vi "poly_recursive_set_cluster_element(s).vi"(6 "stop after 1st one?":bool, 7 "delimiter (/)":string="/", 8 "error in (no error)":errorcluster, 9 "field name":string, 10 "Data":variant, 11 "Cluster":variant) -> (0 "error out":errorcluster, 2 "set?":bool, 3 "Cluster out":variant)   [LabVIEW 2015]
uses:
  <vilib>/Utility/Data Type/NI_Data Type.lvlib
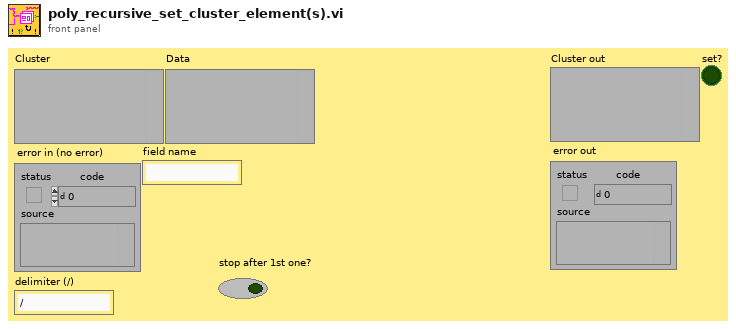
[diagram p1: front panel]
types:
  T1 = typedef "NI_Data Type.lvlib/Data Type.ctl" = enum8{"Invalid Type", "Void", "I8", "I16", "I32", "I64", "U8", "U16", "U32", "U64", "Single Float", "Double Float", "Extended Float", "Single Complex", "Double Complex", "Extended Complex", "Enum U8", "Enum U16", "Enum U32", "Enum U64", "Single Float With Unit", "Double Float With Unit", "Extended Float With Unit", "Single Complex with Unit", "Double Complex with Unit", "Extended Complex with Unit", "Boolean", "String", "Path", "Picture", "Tag", "Array", "Cluster", "Variant", "LV Variant", "Waveform", "Timestamp", "Digital Waveform", "Digital Data", "ExpressData", "Refnum", "External Data", "VI", "Poly VI", "LabVIEW Class Instance", "Fixed Point"}
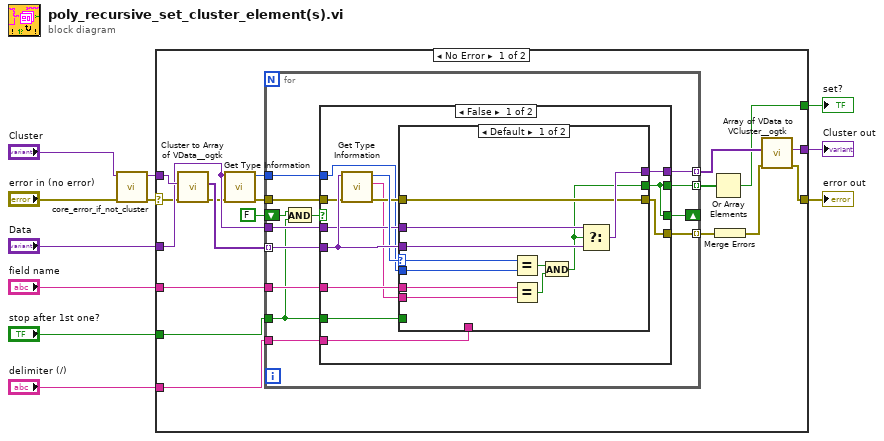
[diagram p0: block diagram]
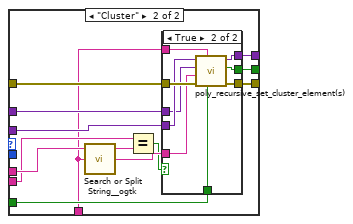
[diagram p2: hidden frame]
diagram:
  n1 = call "core_error_if_not_cluster.vi"("Error in"="error in (no error)", "Cluster"="Cluster") -> ("Error out"=w4:errorcluster, "Cluster duplicate"=w2:variant)  [unwired: 8 in]
  n2 = case shown="No Error" w4 {
    selector: w4 -> [w15 w94]
    tunnel: w2 -> [w28 _]
    tunnel: [w26 _] -> w11
    tunnel: "Data" -> [w17 _]
    tunnel: [w23 w94] -> w9
    tunnel: "field name" -> [w22 _]
    tunnel: [w20 _] -> w7
    tunnel: "stop after 1st one?" -> [w19 _]
    tunnel: "delimiter (/)" -> [w12 _]
    frame No Error {
      n3 = call <userlib>:"Cluster to Array of VData__ogtk.vi"("error in (no error)"=w15, "Cluster"=w28) -> ("error out"=w14:errorcluster, "Array of VData"=w29:variant[])  [unwired: 8 in]
      n4 = call <vilib>:"Get Type Information.vi"("error in (no error)"=w14, "Variant"=w17) -> ("error out"=w13:errorcluster, "Type"=w16:T1)  [unwired: 5 in, 3 out]
      n5 = for {
        tunnel: w29 -> [w41] mode=indexing
        tunnel: [w42] -> w27 mode=indexing
        tunnel: w17 -> [w40]
        tunnel: [w38] -> w25 mode=indexing
        tunnel: w13 -> [w39]
        tunnel: w22 -> [w37]
        tunnel: [w32] -> w21 mode=indexing
        shift-right: [w36] -> _
        shift-left: FALSE ("set?") -> [w34]
        tunnel: w19 -> [w31]
        tunnel: w16 -> [w35]
        tunnel: w12 -> [w30]
        n6 = And(x=w34, y=w31) -> (x .and. y?=w33:bool)
        n7 = case shown="False" w33 {
          selector: w33 -> [_ w92]
          tunnel: [w55 w91] -> w42
          tunnel: w41 -> [w54 w91]
          tunnel: w40 -> [w52 _]
          tunnel: w39 -> [w51 w93]
          tunnel: [w49 w93] -> w38
          tunnel: w37 -> [w48 _]
          tunnel: [w45 w92] -> w36
          tunnel: w35 -> [w46 _]
          tunnel: [w45 _] -> w32
          tunnel: w31 -> [w44 _]
          tunnel: w30 -> [w43 _]
          frame False {
            n8 = call <vilib>:"Get Type Information.vi"("error in (no error)"=w51, "Variant"=w54) -> ("error out"=w50:errorcluster, "Name"=w47:string, "Type"=w53:T1)  [unwired: 5 in, 2 out]
            n9 = case shown="Default" w53 {
              selector: w53 -> [w59 _]
              tunnel: [w66 w75] -> w55
              tunnel: w54 -> [w63 w77]
              tunnel: w52 -> [w64 w76]
              tunnel: w50 -> [w65 w79]
              tunnel: [w65 w78] -> w49
              tunnel: w48 -> [w62 w74]
              tunnel: w47 -> [w58 w72]
              tunnel: [w61 w69] -> w45
              tunnel: w46 -> [w60 _]
              tunnel: w44 -> [_ w68]
              tunnel: w43 -> [_ w67]
              frame Default {
                n10 = Equal?(x=w59, y=w60) -> (x = y?=w57:bool)
                n11 = Equal?(x=w62, y=w58) -> (x = y?=w56:bool)
                n12 = And(x=w57, y=w56) -> (x .and. y?=w61:bool)
                n13 = Select(t=w64, s=w61, f=w63) -> (s? t:f=w66:variant)
              }
              frame "Cluster" {
                n14 = call <userlib>:"Search or Split String__ogtk.vi"("search string/char (-)"=w67, "string"=w74) -> ("substring after match"=w73:string, "substring before match"=w71:string)  [unwired: 1 in, 1 out]
                n15 = Equal?(x=w72, y=w71) -> (x = y?=w70:bool)
                n16 = case shown="True" w70 {
                  tunnel: w79 -> [w80 w90]
                  tunnel: [w80 w89] -> w78
                  tunnel: w77 -> [w81 w88]
                  tunnel: w76 -> [_ w87]
                  tunnel: [w81 w86] -> w75
                  tunnel: w73 -> [_ w85]
                  tunnel: [_ w84] -> w69
                  tunnel: w68 -> [_ w83]
                  tunnel: w67 -> [_ w82]
                  frame False {
                  }
                  frame True {
                    n17 = call "poly_recursive_set_cluster_element(s).vi"("stop after 1st one?"=w83, "delimiter (/)"=w82, "error in (no error)"=w90, "field name"=w85, "Data"=w87, "Cluster"=w88) -> ("error out"=w89:errorcluster, "set?"=w84:bool, "Cluster out"=w86:variant)  [unwired: 3 in]
                  }
                }
              }
            }
          }
          frame True {
          }
        }
      }
      n18 = Or Array Elements(Boolean array=w21) -> (logical OR=w20:bool)
      n19 = Merge Errors(w25) -> (w24:errorcluster)
      n20 = call <userlib>:"Array of VData to VCluster__ogtk.vi"("error in (no error)"=w24, "Array"=w27) -> ("error out"=w23:errorcluster, "VCluster"=w26:variant)  [unwired: 8 in]
    }
    frame Error {
    }
  }
  "Cluster out" <- w11
  "error out" <- w9
  "set?" <- w7
